vi "PID Straight.vi"(6 "Reinitialize":bool, 8 "Error In":errorcluster, 9 "Gyro Angle":dbl, 10 "Current Distance":dbl, 11 "Target Distance":dbl) -> (0 "Error Out":errorcluster, 2 "Right Power":dbl, 3 "Left Power":dbl)   [LabVIEW 2016]
uses:
  <vilib>/addons/control/pid/pid.llb/PID (DBL).vi
  <vilib>/addons/control/pid/NI_PID_pid.lvlib
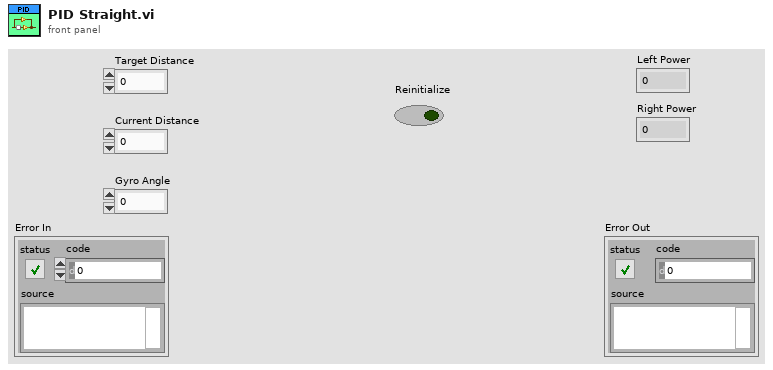
[diagram p1: front panel]
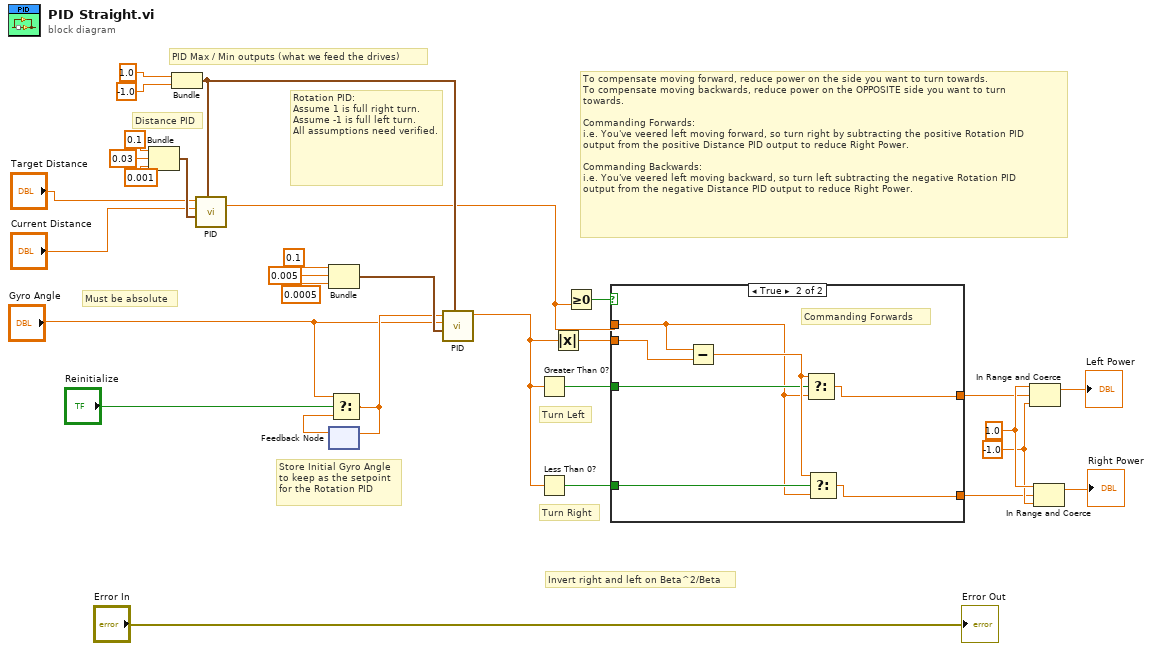
[diagram p0: block diagram]
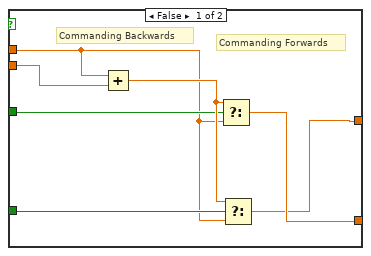
[diagram p2: hidden frame]
diagram:
  w13 = -1.0
  w14 = 1.0
  # "Invert right and left on Beta^2/Beta"
  # "Turn Right"
  # "Turn Left"
  # "To compensate moving forward, reduce power on the side you want to turn towards.\nTo compensate moving backwards, reduce power on the OPPOSITE side you want to turn\ntowards.\n\nCommanding Forwards:\ni.e. You've veered left moving forward, so turn right by subtracting the positive Rotation PID\noutput from the positive Distance PID output to reduce Right Power.\n\nCommanding Backwards:\ni.e. You've veered left moving backward, so turn left subtracting the negative Rotation PID \noutput from the negative Distance PID output to reduce Right Power."
  # "PID Max / Min outputs (what we feed the drives)"
  # "Must be absolute"
  # "Rotation PID:\nAssume 1 is full right turn.\nAssume -1 is full left turn.\nAll assumptions need verified."
  # "Distance PID"
  # "Store Initial Gyro Angle\nto keep as the setpoint\nfor the Rotation PID"
  n1 = Bundle(0.1, 0.03, 0.001) -> (w25:cluster{dbl, dbl, dbl})  [unwired: 1 in]
  n2 = Bundle(1.0, -1.0) -> (w18:cluster{dbl, dbl})  [unwired: 1 in]
  n3 = call-poly <vilib>:"PID.vi"("output range"=w18, "PID gains"=w25, "process variable"="Current Distance", "setpoint"="Target Distance") -> ("output"=w12:dbl)  [unwired: 6 in, 1 out]
  n4 = Bundle(0.1, 0.005, 0.0005) -> (w19:cluster{dbl, dbl, dbl})  [unwired: 1 in]
  n5 = feedback #1() -> (w4:dbl)  [unwired: 1 in]
  n6 = Select(t="Gyro Angle", s="Reinitialize", f=w4) -> (s? t:f=w2:dbl)
  n7 = feedback-in #1(w2) -> ()
  n8 = call-poly <vilib>:"PID.vi"("output range"=w18, "PID gains"=w19, "process variable"="Gyro Angle", "setpoint"=w2) -> ("output"=w6:dbl)  [unwired: 6 in, 1 out]
  n9 = Greater Than 0?(x=w6) -> (x > 0?=w8:bool)
  n10 = Less Than 0?(x=w6) -> (x < 0?=w7:bool)
  n11 = Absolute Value(x=w6) -> (abs(x)=w11:dbl)
  n12 = Greater Or Equal To 0?(x=w12) -> (x >= 0?=w17:bool)
  n13 = case shown="True" w17 {
    tunnel: w11 -> [w34 w44]
    tunnel: w12 -> [w31 w38]
    tunnel: [w33 w42] -> w10
    tunnel: [w32 w41] -> w9
    tunnel: w8 -> [w36 w40]
    tunnel: w7 -> [w35 w39]
    frame False {
      # "Commanding Forwards"
      # "Commanding Backwards"
      n14 = Add(x=w31, y=w34) -> (x+y=w37:dbl)
      n15 = Select(t=w37, s=w36, f=w31) -> (s? t:f=w33:dbl)
      n16 = Select(t=w37, s=w35, f=w31) -> (s? t:f=w32:dbl)
    }
    frame True {
      # "Commanding Forwards"
      n17 = Subtract(x=w38, y=w44) -> (x-y=w43:dbl)
      n18 = Select(t=w43, s=w40, f=w38) -> (s? t:f=w41:dbl)
      n19 = Select(t=w43, s=w39, f=w38) -> (s? t:f=w42:dbl)
    }
  }
  n20 = In Range and Coerce(upper limit=w14, x=w9, lower limit=w13) -> (coerced(x)=→"Left Power":dbl)  [unwired: 1 out]
  n21 = In Range and Coerce(upper limit=w14, x=w10, lower limit=w13) -> (coerced(x)=→"Right Power":dbl)  [unwired: 1 out]
  "Error Out" <- "Error In"
